vi "worksheet insert image buffer opt.vi"(5 "options":T1, 6 "image_size":u32, 7 "image_buffer":string, 8 "error in (no error)":errorcluster, 9 "col":u16, 10 "row":u32, 11 "worksheet":u32) -> (0 "error out":errorcluster, 2 "function return":u32(ring), 3 "options out":T1)   [LabVIEW 8.6]
doc: "lxw_error worksheet_insert_image_buffer_opt(lxw_worksheet worksheet, lxw_row_t row, lxw_col_t col, const unsigned char *image_buffer, size_t image_size, lxw_image_options *options);"
uses:
  pending_lvxlsxwriter/xlsxwriter.dll
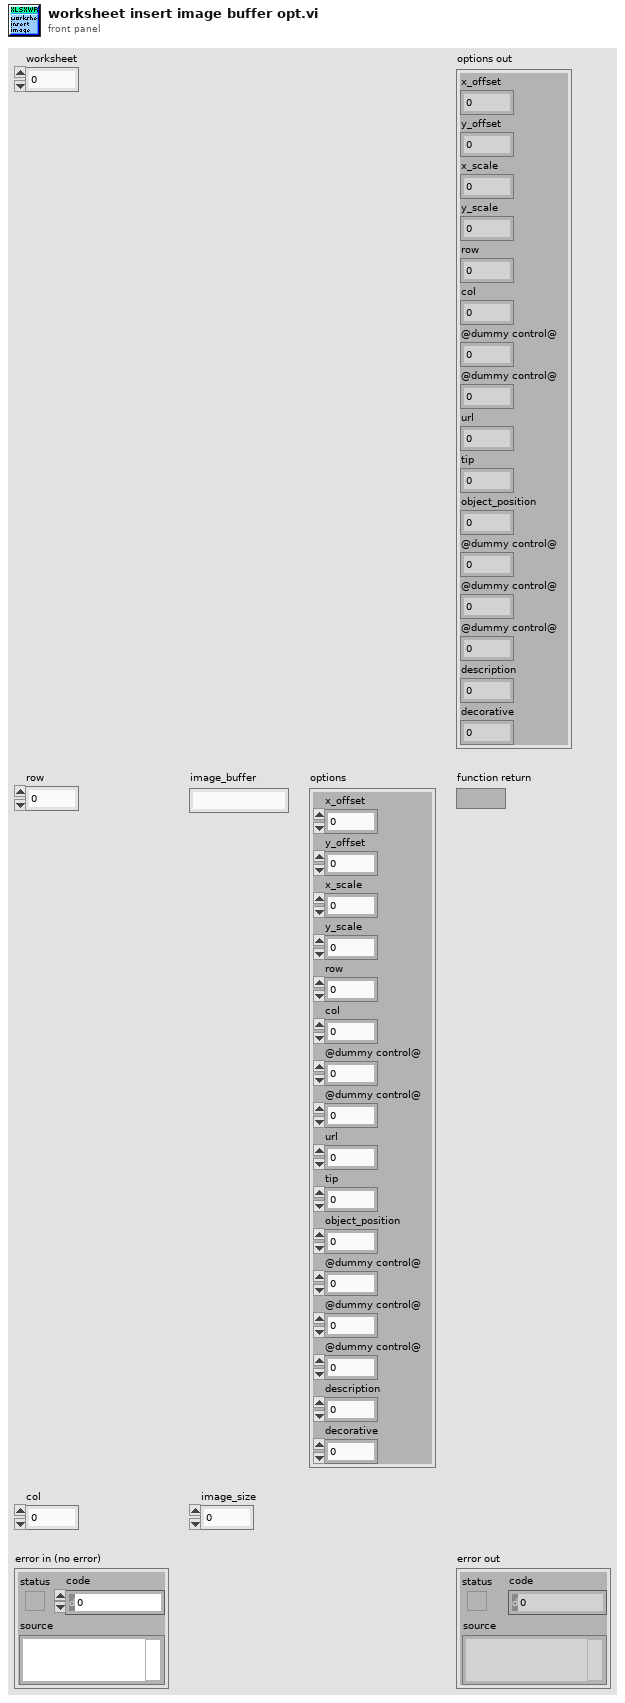
[diagram p1: front panel]
types:
  T1 = cluster{"x_offset":i32, "y_offset":i32, "x_scale":dbl, "y_scale":dbl, "row":u32, "col":u16, "@dummy control@":i8, "@dummy control@":i8, "url":u32, "tip":u32, "object_position":u8, "@dummy control@":i8, "@dummy control@":i8, "@dummy control@":i8, "description":u32, "decorative":u32}
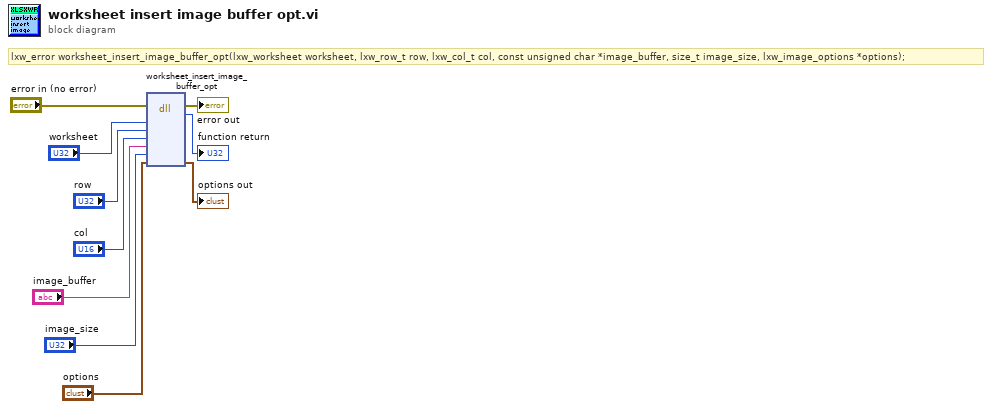
[diagram p0: block diagram]
diagram:
  # "lxw_error worksheet_insert_image_buffer_opt(lxw_worksheet worksheet, lxw_row_t row, lxw_col_t col, const unsigned char *image_buffer, size_t image_size, lxw_image_options *options);"
  n1 = dll-call lib="C:/Users/WDAGUtilityAccount/Desktop/pending_lvxlsxwriter/xlsxwriter.*" fn="worksheet_insert_image_buffer_opt"(error in="error in (no error)", "worksheet"="worksheet", "row"="row", "col"="col", "image_buffer"="image_buffer", "image_size"="image_size", "options"="options") -> (error out=→"error out":errorcluster, →"function return":u32, "options"=→"options out":T1)  [unwired: 7 in, 1 out]
